vi "PMOD Example(FPGA).vi"() -> ()   [LabVIEW 2014]
uses:
  <vilib>/Platform/TimedLoop/XDataNode/XDataNode.xnode
  <vilib>/Platform/TimedLoop/XDataNode/nitl_modes.ctl
  <vilib>/Platform/TimedLoop/XDataNode/XDNodeRunTimeDep.lvlib
  <vilib>/Platform/TimedLoop/XDataNode/wakeup.ctl
  <vilib>/Platform/TimedLoop/XDataNode/timing_clust.ctl
  SPIAPI/DIO/SPI Digital IO Lines.ctl
  <vilib>/SPI API/SPIAPI/DIO/SPI DIO Enable Lines.ctl
  <userlib>/_NI SPI IP/FPGA/Controllers/Public/Spi Master Outputs.ctl
  <userlib>/_NI SPI IP/FPGA/Controllers/NI SPI IP FPGA.lvlib
  <userlib>/_NI SPI IP/FPGA/Controllers/Public/Transfer Settings.ctl
panel:
  out "Raw ADC Data":u64
  out "read Iterations":i32
  in  "Data To ADC":u64=2147483648
  in  "Chip Select":u8
  in  "SPI PHY Settings":T1={"Divide Value"=20, "Transfer Length (bits)"=32, "CS Asserted Polarity"=FALSE, "Clock Polarity (CPOL)"=FALSE, "Clock Phase (CPHA)"=FALSE, "Lengthen MISO Setup"=FALSE, "Direction Change Bit"=0, "MOSI Starts as Output"=FALSE, "Tristatable MOSI"=FALSE} {"Direction Change Bit" max=64 step=1; "Transfer Length (bits)" min=1 max=64 step=1}
  out "spi output":T2
  in  "data rate (S/s)":u32=10000
  out "oclk freq":u32
  out "oclk div":u32
  out "FPGA Error":errorcluster
  out "Acq Loop Ticks":u32
  # "OUTPUT"
  # "INPUT"
  # "ADC Data::Debug"
  # "Acquisition Parameters"
  # "SPI PHY Settings"
  # "Debug"
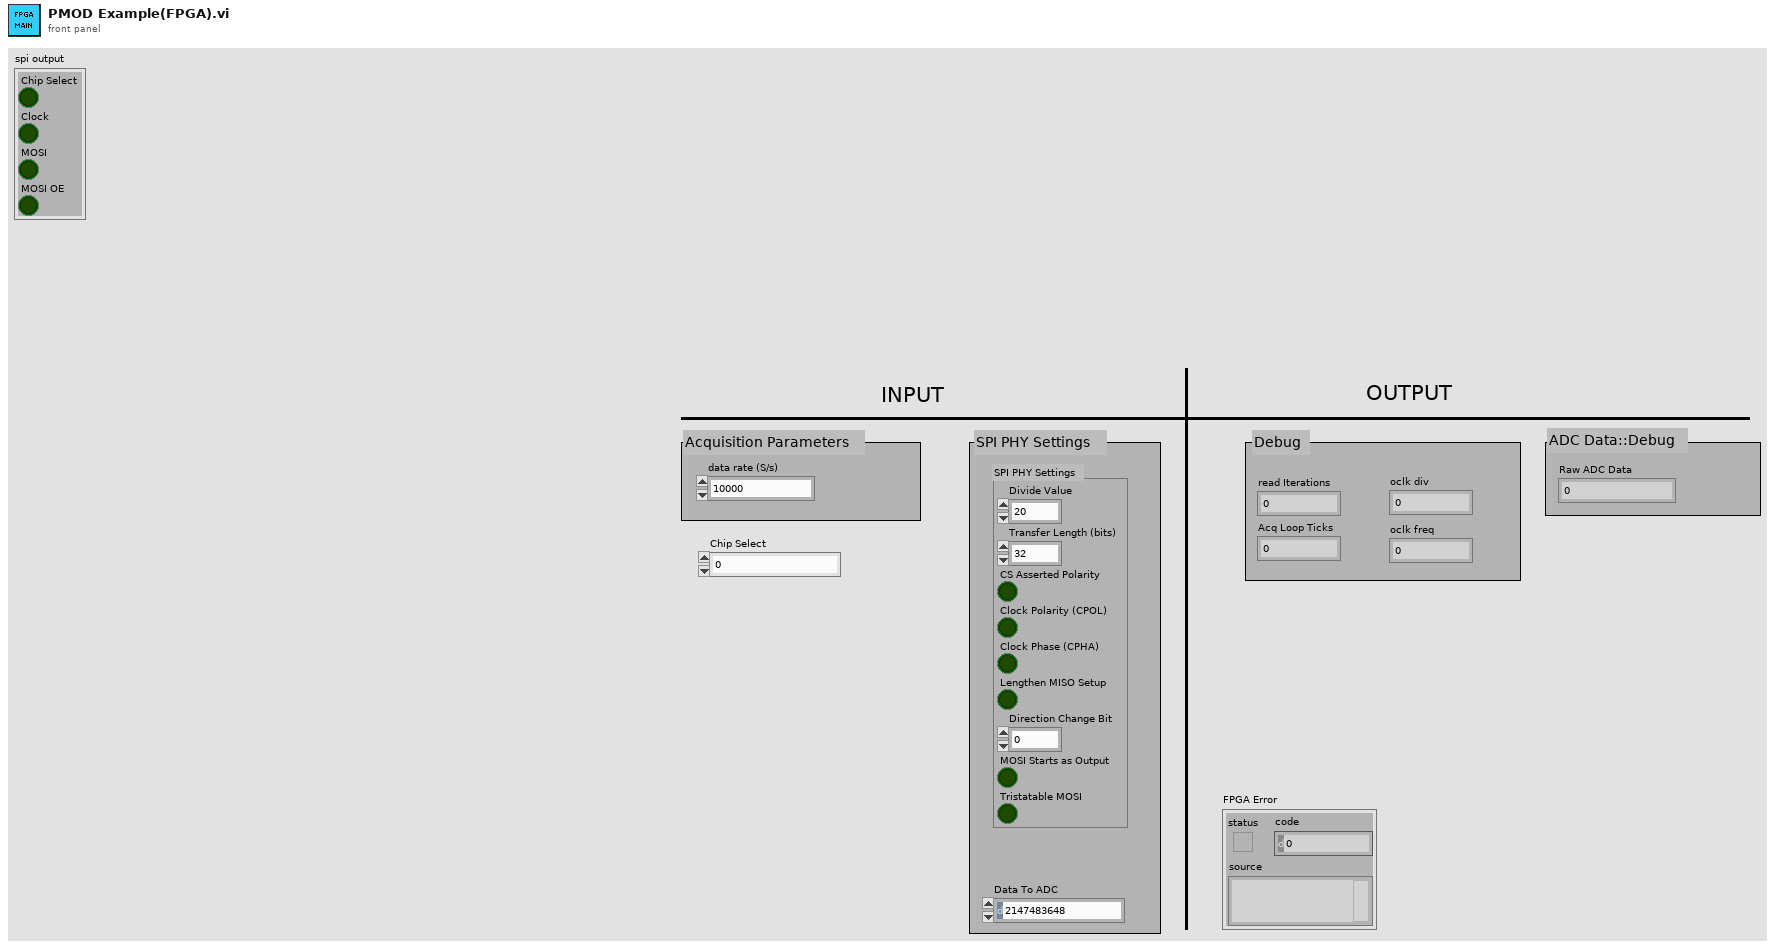
[diagram p1: front panel]
types:
  T1 = typedef "NI SPI IP FPGA.lvlib/Transfer Settings.ctl" = cluster{"Divide Value":u8, "Transfer Length (bits)":u8, "CS Asserted Polarity":bool, "Clock Polarity (CPOL)":bool, "Clock Phase (CPHA)":bool, "Lengthen MISO Setup":bool, "Direction Change Bit":u8, "MOSI Starts as Output":bool, "Tristatable MOSI":bool}
  T2 = typedef "NI SPI IP FPGA.lvlib/Spi Master Outputs.ctl" = cluster{"Chip Select":bool, "Clock":bool, "MOSI":bool, "MOSI OE":bool}
  T3 = typedef "SPI Digital IO Lines.ctl" = cluster{"SCLK":refnum<k21>, "MISO":refnum<k21>, "MOSI":refnum<k21>, "CS 0":refnum<k21>, "CS 1":refnum<k21>, "CS 2":refnum<k21>, "CS 3":refnum<k21>, "CS 4":refnum<k21>, "CS 5":refnum<k21>}
  T4 = typedef "SPI DIO Enable Lines.ctl" = cluster{"SCLK_en":refnum<k21>, "MISO_en":refnum<k21>, "MOSI_en":refnum<k21>, "CS0_en":refnum<k21>, "CS1_en":refnum<k21>, "CS2_en":refnum<k21>, "CS3_en":refnum<k21>, "CS4_en":refnum<k21>, "CS5_en":refnum<k21>}
  T5 = typedef "Internal Data (SPI API).ctl" = cluster{"DLU To SPI Engine Data FIFO":refnum<k21>, "SPI Engine to DLU Data FIFO":refnum<k21>, "Data to SPI Engine (Cache) Register":refnum<k21>, "SPI PHY Settings to SPI Engine (Cahche) Register":refnum<k21>}
  T6 = typedef "XDNodeRunTimeDep.lvlib/timing_clust.ctl" = cluster{"Expected End [f-1]":u64, "Actual End [f-1]":u64, "Finished Late? [f-1]":bool, "Expected End [i-1]":u64, "Actual End [i-1]":u64, "Finished Late? [i-1]":bool, "Expected Start [i]":u64, "Actual Start [i]":u64, "Expected Start [f]":u64, "Actual Start [f]":u64, "Source Name":string, "Structure Name":string, "Period":i64, "Deadline":i64, "Offset":i64, "Start":i64, "Priority":i32, "Timeout":i32, "Mode":T7, "Wakeup Reason":T8, "Error":errorcluster, "Source Type":string, "Secondary Source Type":string, "Global End Time":u64, "Global Start Time":u64, "Frame Duration":u64, "Iteration Duration":u64, "Assigned CPU":i32, "I/O Scan Engine Mode":u32}
  T7 = typedef "XDNodeRunTimeDep.lvlib/nitl_modes.ctl" = enum32{"No Change", "Process missed periods, maintain original phase", "Discard missed periods, maintain original phase", "Process missed periods, ignore original phase", "Discard missed periods, ignore original phase"}
  T8 = typedef "XDNodeRunTimeDep.lvlib/wakeup.ctl" = enum32{"Normal", "Aborted", "Asynchronous wakeup", "Timing source error", "Timed loop error", "Timeout"}
  T9 = typedef "SPI Response Information.ctl" = cluster{"Data to Node":u64, "Node Id":u16}
  T10 = typedef "NI SPI IP FPGA.lvlib/Spi Master Inputs.ctl" = cluster{"MISO":bool}
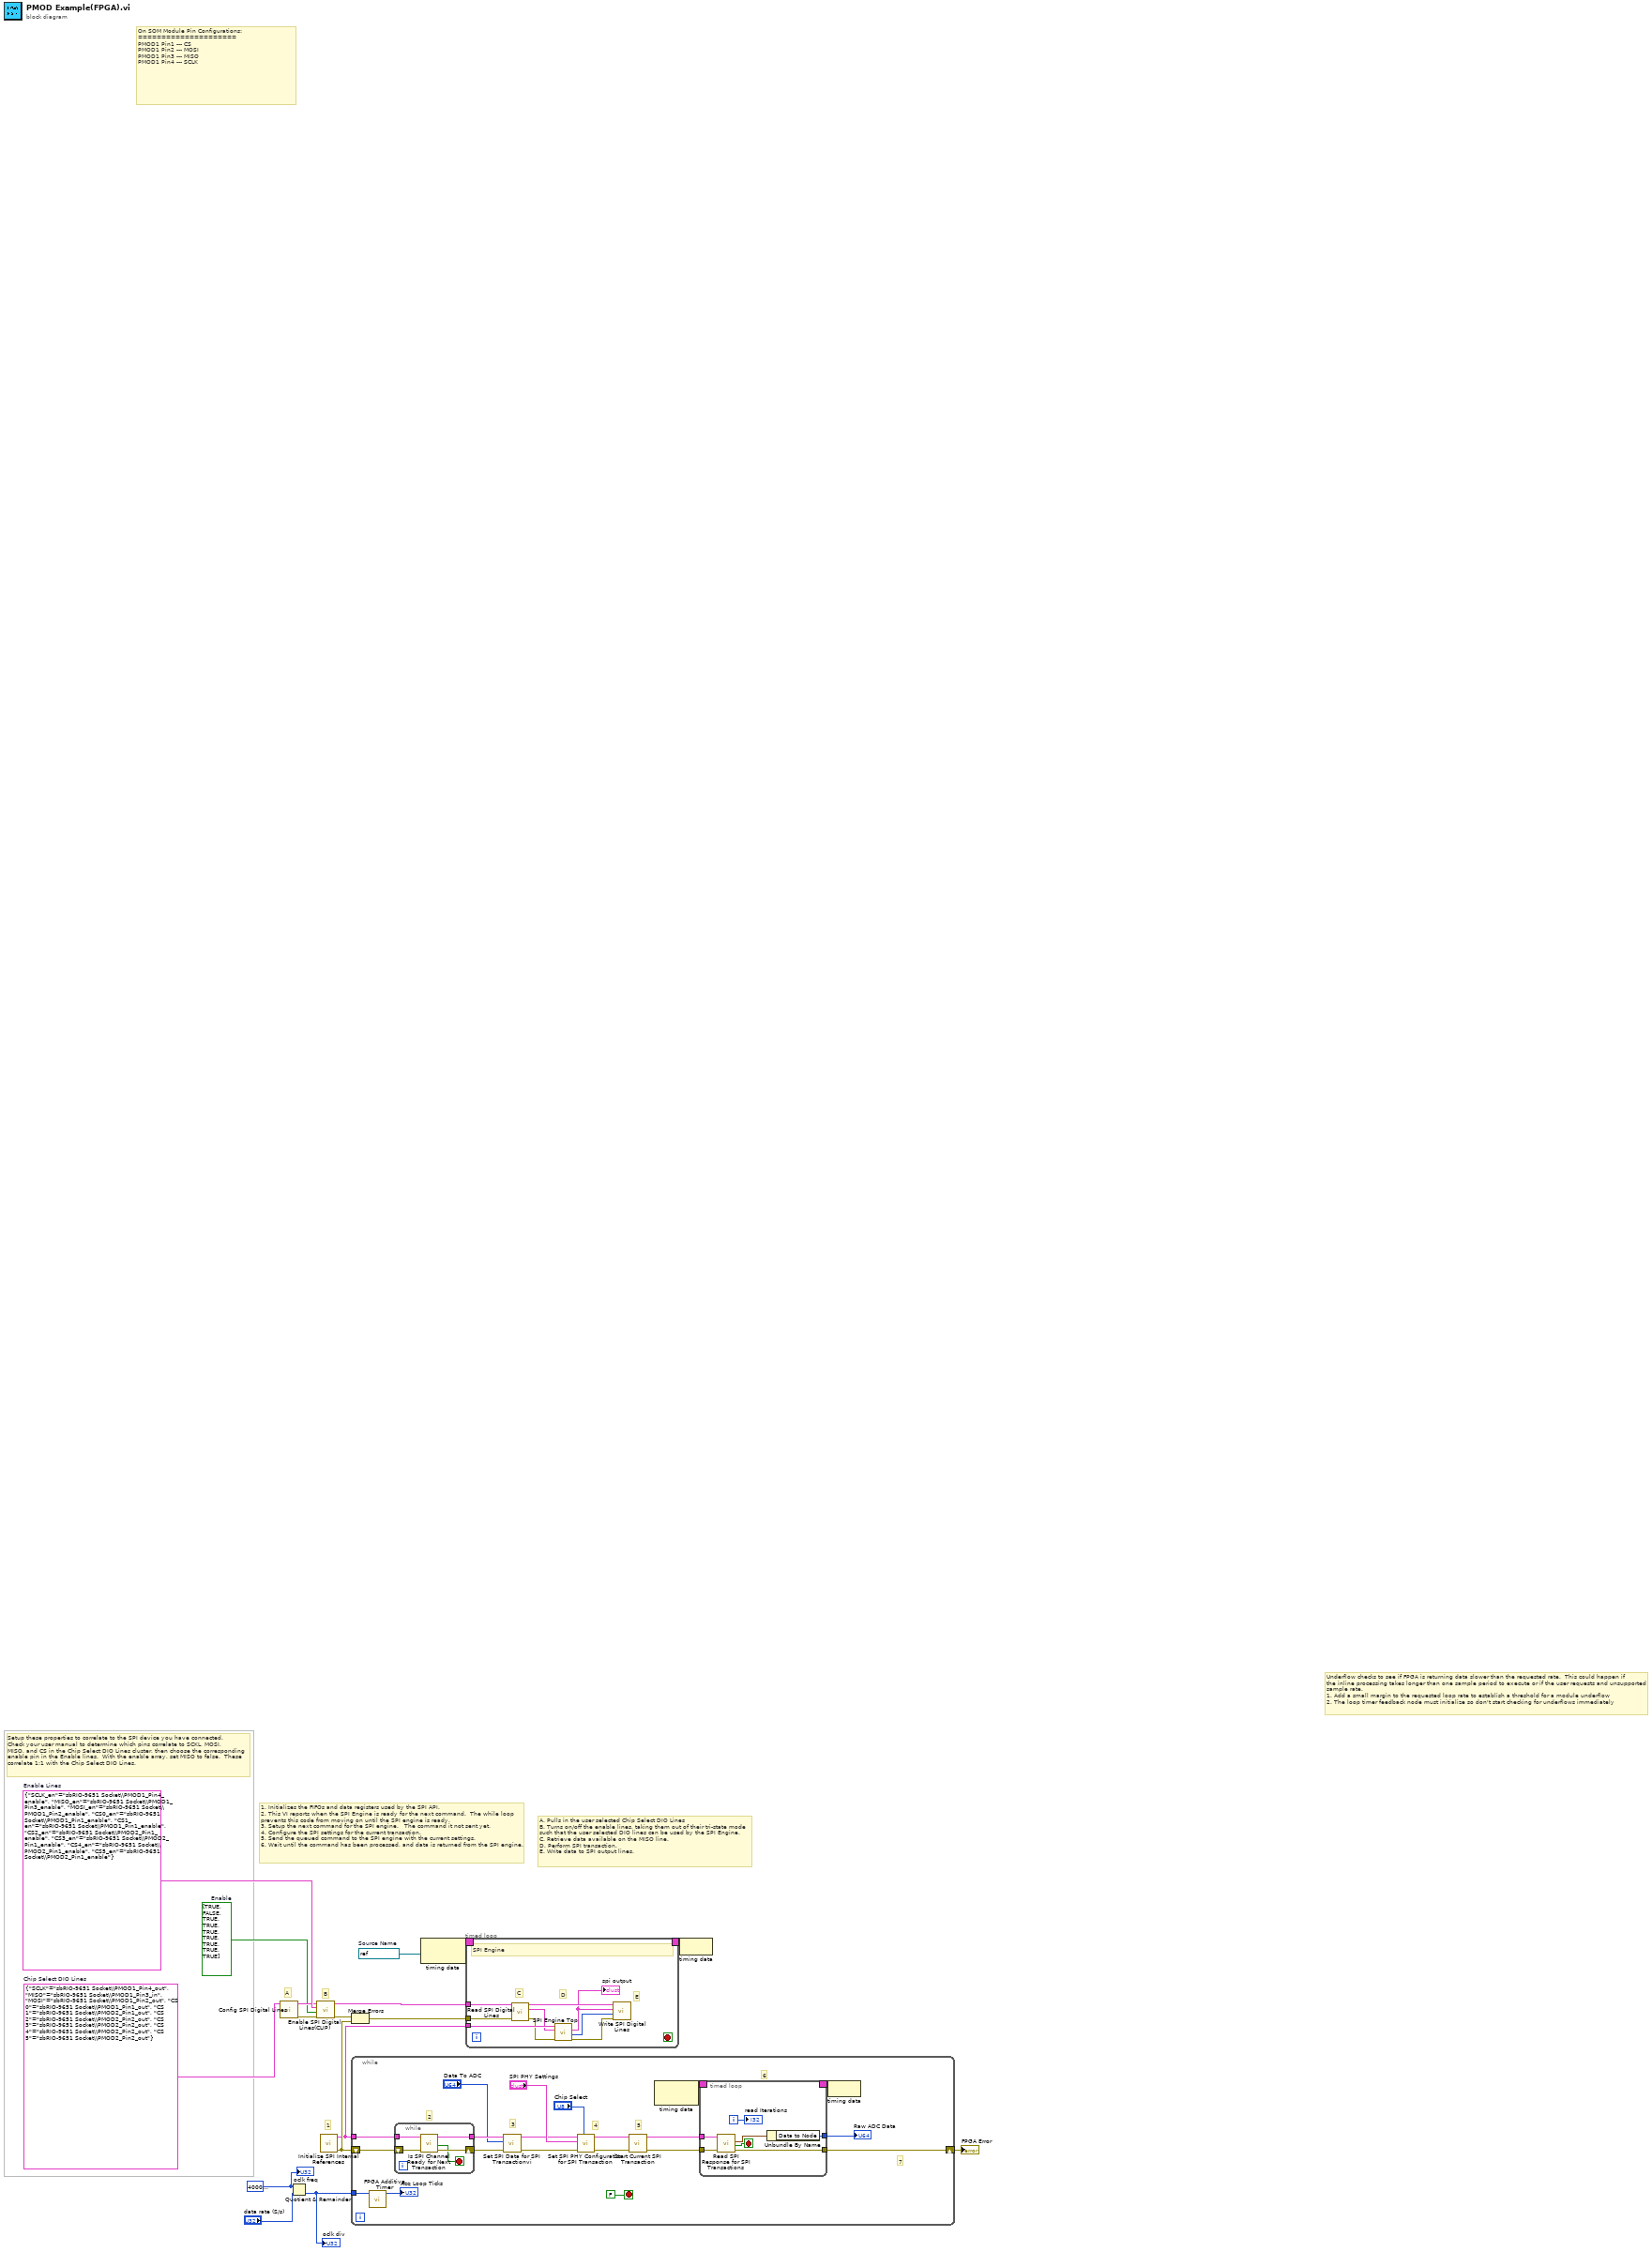
[diagram p0: block diagram]
diagram:
  w2 = T3 {"SCLK"="sbRIO-9651 Socket\\PMOD1_Pin4_out", "MISO"="sbRIO-9651 Socket\\PMOD1_Pin3_in", "MOSI"="sbRIO-9651 Socket\\PMOD1_Pin2_out", "CS 0"="sbRIO-9651 Socket\\PMOD1_Pin1_out", "CS 1"="sbRIO-9651 Socket\\PMOD2_Pin1_out", "CS 2"="sbRIO-9651 Socket\\PMOD2_Pin2_out", "CS 3"="sbRIO-9651 Socket\\PMOD2_Pin2_out", "CS 4"="sbRIO-9651 Socket\\PMOD2_Pin2_out", "CS 5"="sbRIO-9651 Socket\\PMOD2_Pin2_out"}  # Chip Select DIO Lines
  w3 = bool[] [TRUE, FALSE, TRUE, TRUE, TRUE, TRUE, TRUE, TRUE, TRUE]  # Enable
  w8 = refnum<k21> "120MHz"  # Source Name
  w12 = u32 40000000 ("oclk freq")
  w17 = T4 {"SCLK_en"="sbRIO-9651 Socket\\PMOD1_Pin4_enable", "MISO_en"="sbRIO-9651 Socket\\PMOD1_Pin3_enable", "MOSI_en"="sbRIO-9651 Socket\\PMOD1_Pin2_enable", "CS0_en"="sbRIO-9651 Socket\\PMOD1_Pin1_enable", "CS1_en"="sbRIO-9651 Socket\\PMOD1_Pin1_enable", "CS2_en"="sbRIO-9651 Socket\\PMOD2_Pin1_enable", "CS3_en"="sbRIO-9651 Socket\\PMOD2_Pin1_enable", "CS4_en"="sbRIO-9651 Socket\\PMOD2_Pin1_enable", "CS5_en"="sbRIO-9651 Socket\\PMOD2_Pin1_enable"}  # Enable Lines
  # "A. Pulls in the user selected Chip Select DIO Lines\nB. Turns on/off the enable lines, taking them out of their tri-state mode \nsuch that the user selected DIO lines can be used by the SPI Engine.\nC. Retrieve data available on the MISO line.\nD. Perform SPI transaction.\nE. Write data to SPI output lines."
  # "B"
  # "A"
  # "1. Initializes the FIFOs and data registers used by the SPI API.\n2. This VI reports when the SPI Engine is ready for the next command.  The while loop \nprevents this code from moving on until the SPI engine is ready.\n3. Setup the next command for the SPI engine.   The command it not sent yet.\n4. Configure the SPI settings for the current transaction.\n5. Send the queued command to the SPI engine with the current settings.\n6. Wait until the command has been processed, and data is returned from the SPI engine."
  # "1"
  # "Setup these properties to correlate to the SPI device you have connected.\nCheck your user manual to determine which pins correlate to SCKL, MOSI,\nMISO, and CS in the Chip Select DIO Lines cluster, then choose the corresponding\nenable pin in the Enable lines.  With the enable array, set MISO to false.  These\ncorrelate 1:1 with the Chip Select DIO Lines."
  # "On SOM Module Pin Configurations:\n=====================\nPMOD1 Pin1 --- CS\nPMOD1 Pin2 --- MOSI\nPMOD1 Pin3 --- MISO\nPMOD1 Pin4 --- SCLK"
  # "Underflow checks to see if FPGA is returning data slower than the requested rate.  This could happen if\nthe inline processing takes longer than one sample period to execute or if the user requests and unsupported\nsample rate.\n1. Add a small margin to the requested loop rate to establish a threshold for a module underflow \n2. The loop timer feedback node must initialize so don't start checking for underflows immediately"
  n1 = call <vilib>:"Config SPI Digital Lines.vi"("SPI DIO Lines"=w2) -> ("error out"=w4:errorcluster, "Chip Select DIO Lines"=w5:T3)  [unwired: 9 in]
  n2 = Quotient & Remainder(x=w12, y="data rate (S/s)") -> (floor(x/y)=w14:u32)  [unwired: 1 out]
  "oclk div" <- w14
  n3 = call <vilib>:"Enable SPI Digital Lines(CLIP).vi"("error in"=w4, "Enable"=w3, "Enable Lines"=w17, "SPI DIO Lines"=w5) -> ("error out"=w6:errorcluster, "Chip Select DIO Lines"=w7:T3)  [unwired: 6 in]
  n4 = call "Initialize SPI Internal References.vi"() -> ("error out"=w11:errorcluster, "SPI API References"=w10:T5)  [unwired: 10 in]
  n5 = Merge Errors(w6, w11) -> (w9:errorcluster)
  n6 = while {
    tunnel: w14 -> [w37]
    shift-right: [w19] -> w1
    shift-left: w11 -> [w32]
    tunnel: w10 -> [w33]
    stop <- FALSE stop-if-true
    # "7"
    # "6"
    # "5"
    # "4"
    # "3"
    # "2"
    n7 = call "FPGA Additive Timer.vi"("Numeric in"=w37) -> ("Numeric out"=→"Acq Loop Ticks":u32)  [unwired: 10 in]
    n8 = while {
      shift-right: [w42] -> w35
      shift-left: w32 -> [w39]
      tunnel: w33 -> [w40]
      tunnel: [w41] -> w34
      stop <- w38 stop-if-true
      n9 = call "Is SPI Channel Ready for Next Transaction.vi"("error in"=w39, "Private Data In"=w40) -> ("error out"=w42:errorcluster, "SPI Channel Ready"=w38:bool, "Private Data Out"=w41:T5)  [unwired: 6 in, 1 out]
    }
    n10 = call "Set SPI Data for SPI Transactionvi.vi"("error in"=w35, "Data In"="Data To ADC", "Private Data In"=w34) -> ("error out"=w26:errorcluster, "Private Data Out"=w27:T5)  [unwired: 7 in]
    n11 = call "Set SPI PHY Configuration for SPI Transaction.vi"("Chip Select"="Chip Select", "error in"=w26, "SPI PHY Settings"="SPI PHY Settings", "Private Data In"=w27) -> ("error out"=w23:errorcluster, "Private Data Out"=w24:T5)  [unwired: 6 in]
    n12 = call "Start Current SPI Transaction.vi"("error in"=w23, "Private Data In"=w24) -> ("error out"=w28:errorcluster, "Private Data Out"=w22:T5)  [unwired: 7 in, 1 out]
    n13 = node-c288() -> (w31:T6)  [unwired: 1 in]
    n14 = timed-loop {
      timing: w31 -> [_]
      timing-out: [_] -> w30
      tunnel: w28 -> [w49]
      tunnel: w22 -> [w48]
      tunnel: [w43] -> w18
      tunnel: [w45] -> w19
      i -> [w44]
      stop <- w47 stop-if-true
      n15 = call "Read SPI Response for SPI Transactions.vi"("error in"=w49, "Private Data In"=w48) -> ("error out"=w45:errorcluster, "Read Data Valid?"=w47:bool, "Read Data"=w46:T9)  [unwired: 6 in, 1 out]
      n16 = Unbundle By Name(w46) -> ("Data to Node"=w43:u64)
      "read Iterations" <- w44
    }
    "Raw ADC Data" <- w18
    n17 = node-c288(w30) -> ()
  }
  "FPGA Error" <- w1
  n18 = node-c288(w8) -> (w16:T6)
  n19 = timed-loop {
    tunnel: w10 -> [w59]
    tunnel: w9 -> [w57]
    tunnel: w7 -> [w61]
    timing: w16 -> [_]
    timing-out: [_] -> w15
    stop <- _ stop-if-true
    # "E"
    # "D"
    # "C"
    # "SPI Engine"
    n20 = call "Read SPI Digital Lines.vi"("Chip Select DIO Lines"=w61, "error in"=w57) -> ("Chip Select DIO Lines Out"=w62:T3, "SPI Read Data"=w58:T10, "error out"=w56:errorcluster)  [unwired: 11 in]
    n21 = call "SPI Engine Top.vi"("error in"=w56, "SPI Read Data"=w58, "SPI API References"=w59) -> ("error out"=w55:errorcluster, "Chip Select ID"=w54:u8, "SPI DIO Output"=w60:T2)  [unwired: 5 in, 1 out]
    "spi output" <- w60
    n22 = call <vilib>:"Write SPI Digital Lines.vi"("error in"=w55, "CS Index"=w54, "spi output"=w60, "Chip Select DIO Lines"=w62) -> ()  [unwired: 6 in, 2 out]
  }
  n23 = node-c288(w15) -> ()
  "oclk freq" <- w12
